vi "Waveform_Generation2.vi"(10 "input cluster":T2) -> (2 "output cluster":T1)   [LabVIEW 2013]
uses:
  waveforms.ctl
  <vilib>/imath/engines/lvmath2/RunTimeEngine/ErrorHandling/NIMS_Finalize Error.vi
  <vilib>/imath/engines/lvmath2/RunTimeEngine/Managers/WorkSpace/UID Generator.vi
  <vilib>/imath/engines/lvmath2/RunTimeEngine/NodeEndStatement/NIMS_NodeEndStatement_Get Vector.vi
  <instcachedir>/0/NIMS_NodeEndStatement_Get Vector_BE4364D373AE46158CA0B14DEB6F98C8.lvgen/NIMS_NodeEndStatement_Get Vector_BE4364D373AE46158CA0B14DEB6F98C8_001.vi
  <vilib>/imath/engines/lvmath/Functions/Error Handling/MergeErrorsWrapper.vi
  <vilib>/imath/engines/lvmath2/RunTimeEngine/Managers/SymbolTable/Clear UID.vi
  <vilib>/imath/engines/lvmath2/RunTimeEngine/NodeEndStatement/NIMS_NodeEndStatement_Output.vi
  <instcachedir>/0/NIMS_NodeEndStatement_Output_53EC0D466D134D7ABD903AC30B43404B.lvgen/NIMS_NodeEndStatement_Output_53EC0D466D134D7ABD903AC30B43404B_011.vi
  <instcachedir>/0/NIMS_NodeEndStatement_Output_53EC0D466D134D7ABD903AC30B43404B.lvgen/NIMS_NodeEndStatement_Output_53EC0D466D134D7ABD903AC30B43404B_001.vi
  <instcachedir>/0/NIMS_NodeEndStatement_Output_53EC0D466D134D7ABD903AC30B43404B.lvgen/NIMS_NodeEndStatement_Output_53EC0D466D134D7ABD903AC30B43404B_005.vi
  <instcachedir>/0/NIMS_NodeEndStatement_Output_53EC0D466D134D7ABD903AC30B43404B.lvgen/NIMS_NodeEndStatement_Output_53EC0D466D134D7ABD903AC30B43404B_010.vi
  <vilib>/imath/engines/lvmath2/RunTimeEngine/RunTimeType/NIMS_RunTimeType_From StrictType (excl LVString).vi
  <instcachedir>/0/NIMS_RunTimeType_From StrictType (excl LVString)_4DEE718D6EB74582AA20236969C084FC.lvgen/NIMS_RunTimeType_From StrictType (excl LVString)_4DEE718D6EB74582AA20236969C084FC_000.vi
  <vilib>/imath/engines/lvmath2/RunTimeEngine/LocalVariableDefStatement/MC_LocalVariableDefStatement_Display.vi
  <vilib>/imath/engines/lvmath2/RunTimeEngine/BuiltInFunctions/abs/NIMS_abs(signed).vi
  <instcachedir>/0/NIMS_abs(signed)_C4FCB8E6058B49B797C7C8D53CA5F6EC.lvgen/NIMS_abs(signed)_C4FCB8E6058B49B797C7C8D53CA5F6EC_000.vi
  <vilib>/imath/engines/lvmath2/RunTimeEngine/BuiltInFunctions/zeros/NIMS_V=zeros(I32,I32).vi
  <vilib>/imathl/engines/lvmath/Functions/Error Handling/Create Error.vi
  <vilib>/imath/engines/lvmath2/RunTimeEngine/RangeToken/NIMS_Range.vi
  <instcachedir>/0/NIMS_Range_7481B155BEE341ECA0F59DDB444E2C09.lvgen/NIMS_Range_7481B155BEE341ECA0F59DDB444E2C09_000.vi
  <vilib>/imath/engines/lvmath2/RunTimeEngine/BuiltInFunctions/linramp/NIMS_linramp.vi
  <vilib>/imath/engines/lvmath2/RunTimeEngine/BuiltInFunctions/length/NIMS_length(GV).vi
  <instcachedir>/0/NIMS_length(GV)_08A3D13377FD4E4B96F5795FBF3698FA.lvgen/NIMS_length(GV)_08A3D13377FD4E4B96F5795FBF3698FA_000.vi
  <vilib>/imath/engines/lvmath2/RunTimeEngine/BuiltInFunctions/repeatmx/NIMS_repeatmx(GM, I32, I32).vi
  <instcachedir>/0/NIMS_repeatmx(GM, I32, I32)_71D32CAC8D434697AB9DA7B55FCB46E4.lvgen/NIMS_repeatmx(GM, I32, I32)_71D32CAC8D434697AB9DA7B55FCB46E4_000.vi
  <vilib>/imath/engines/lvmath2/RunTimeEngine/RowToken/NIMS_RowToken_M_M.vi
  <instcachedir>/0/NIMS_RowToken_M_M_CBE56BFCE95A4183A980645A330616E9.lvgen/NIMS_RowToken_M_M_CBE56BFCE95A4183A980645A330616E9_004.vi
  <vilib>/imath/engines/lvmath2/RunTimeEngine/ErrorHandling/NIMS_Create Error From Enums.vi
  <vilib>/imath/engines/lvmath2/RunTimeEngine/BuiltInFunctions/length/NIMS_length(GM).vi
  <instcachedir>/0/NIMS_length(GM)_47CEC356FCE0482D9BA47DC61C99F2C7.lvgen/NIMS_length(GM)_47CEC356FCE0482D9BA47DC61C99F2C7_000.vi
  <vilib>/imath/engines/lvmath2/RunTimeEngine/IndexRead/NIMS M(S,R2).vi
  <instcachedir>/0/NIMS M(S,R2)_45730E4D0DB74D118F715F4F99DCE4D7.lvgen/NIMS M(S,R2)_45730E4D0DB74D118F715F4F99DCE4D7_000.vi
  <vilib>/imath/engines/lvmath2/RunTimeSupport/NIMS_Error if Not Equal.vi
  <instcachedir>/0/NIMS_Error if Not Equal_902F5D2649E64F5087A1EF57C55C58AB.lvgen/NIMS_Error if Not Equal_902F5D2649E64F5087A1EF57C55C58AB_001.vi
  <vilib>/imath/engines/lvmath2/RunTimeEngine/IndexRead/NIMS V(V).vi
  <instcachedir>/0/NIMS V(V)_298D9CB7BFEB42B8BC8D9C3C28AE8C70.lvgen/NIMS V(V)_298D9CB7BFEB42B8BC8D9C3C28AE8C70_000.vi
  <vilib>/imath/engines/lvmath2/RunTimeEngine/RowToken/NIMS_RowToken_M_SorRV.vi
  <instcachedir>/0/NIMS_RowToken_M_SorRV_6464340A296F47B6970F468C8541F43A.lvgen/NIMS_RowToken_M_SorRV_6464340A296F47B6970F468C8541F43A_000.vi
  <vilib>/imath/engines/lvmath2/RunTimeEngine/RowToken/NIMS_RowToken_SorRV_M.vi
  <instcachedir>/0/NIMS_RowToken_SorRV_M_D0DD9F47061B415B905C482B8C5C3219.lvgen/NIMS_RowToken_SorRV_M_D0DD9F47061B415B905C482B8C5C3219_000.vi
  <vilib>/imath/engines/lvmath2/RunTimeEngine/ArithmeticOperatorToken/NIMS_ArithmeticOperator_plus.vi
  <instcachedir>/0/NIMS_ArithmeticOperator_plus_8A46DAFC24D445C9B2C97B626139369E.lvgen/NIMS_ArithmeticOperator_plus_8A46DAFC24D445C9B2C97B626139369E_003.vi
  <vilib>/imath/engines/lvmath2/RunTimeEngine/BuiltInFunctions/round/NIMS_round(DBL-S).vi
  <vilib>/imath/engines/lvmath2/RunTimeEngine/BuiltInFunctions/ones/NIMS_V=ones(I32,I32).vi
  <instcachedir>/0/NIMS_repeatmx(GM, I32, I32)_71D32CAC8D434697AB9DA7B55FCB46E4.lvgen/NIMS_repeatmx(GM, I32, I32)_71D32CAC8D434697AB9DA7B55FCB46E4_004.vi
  <instcachedir>/0/NIMS_RowToken_M_M_CBE56BFCE95A4183A980645A330616E9.lvgen/NIMS_RowToken_M_M_CBE56BFCE95A4183A980645A330616E9_005.vi
  <vilib>/imath/engines/lvmath2/RunTimeEngine/RangeToken/NIMS_Range_R2 - Integer.vi
  <instcachedir>/0/NIMS_Range_R2 - Integer_C51C130E5EA5464EA148B28CDAB9615A.lvgen/NIMS_Range_R2 - Integer_C51C130E5EA5464EA148B28CDAB9615A_000.vi
  <vilib>/imath/engines/lvmath2/RunTimeEngine/CommandStatement/MC_CommandStatement_break.vi
  <vilib>/imath/engines/lvmath2/RunTimeEngine/ArithmeticOperatorToken/NIMS_ArithmeticOperator_power(S).vi
  <instcachedir>/0/NIMS_ArithmeticOperator_power(S)_7602F12E697C47D8910FAD43BB85D848.lvgen/NIMS_ArithmeticOperator_power(S)_7602F12E697C47D8910FAD43BB85D848_011.vi
  <instcachedir>/0/NIMS_ArithmeticOperator_plus_8A46DAFC24D445C9B2C97B626139369E.lvgen/NIMS_ArithmeticOperator_plus_8A46DAFC24D445C9B2C97B626139369E_004.vi
  <vilib>/imath/engines/lvmath2/RunTimeEngine/BuiltInFunctions/difference/NIMS_difference(GV,I32).vi
  <instcachedir>/0/NIMS_difference(GV,I32)_DC7351DCBCF840A8AE147F50EC2CE86E.lvgen/NIMS_difference(GV,I32)_DC7351DCBCF840A8AE147F50EC2CE86E_000.vi
  <vilib>/imath/engines/lvmath2/RunTimeEngine/VariableToken/Support/NIMS_Vector Boolean Index to I32 Index.vi
  <vilib>/imath/engines/lvmath2/RunTimeEngine/IndexReplace/NIMS V(V)=V.vi
  <instcachedir>/0/NIMS V(V)=V_320D50C59D214ECA9A3F84A49F4F0CE6.lvgen/NIMS V(V)=V_320D50C59D214ECA9A3F84A49F4F0CE6_000.vi
  <vilib>/imath/engines/lvmath2/RunTimeEngine/IndexRead/NIMS V(R2).vi
  <instcachedir>/0/NIMS V(R2)_C76619605A0E4E9F8B2FA9389712AC47.lvgen/NIMS V(R2)_C76619605A0E4E9F8B2FA9389712AC47_000.vi
  <vilib>/imath/engines/lvmath2/RunTimeEngine/BuiltInFunctions/quadn_trap/NIMS_quadn_trap(GV).vi
  <instcachedir>/0/NIMS_quadn_trap(GV)_FA03A60467B0476FA3B590A5FD2D65B5.lvgen/NIMS_quadn_trap(GV)_FA03A60467B0476FA3B590A5FD2D65B5_000.vi
  <vilib>/imath/engines/lvmath2/RunTimeEngine/IndexReplace/NIMS V(S)=S.vi
  <instcachedir>/0/NIMS V(S)=S_66A18068148B4981A312229A93EA5C06.lvgen/NIMS V(S)=S_66A18068148B4981A312229A93EA5C06_000.vi
  <vilib>/imath/engines/lvmath2/RunTimeEngine/BuiltInFunctions/min/1 input/NIMS_min(RV).vi
  <instcachedir>/0/NIMS_min(RV)_EE2DD3E2888846108C5160A664B67832.lvgen/NIMS_min(RV)_EE2DD3E2888846108C5160A664B67832_000.vi
  <vilib>/imath/engines/lvmath2/RunTimeEngine/IndexReplace/NIMS V(V)=S.vi
  <instcachedir>/0/NIMS V(V)=S_43E6004D39A2403BA86EB2871913A93B.lvgen/NIMS V(V)=S_43E6004D39A2403BA86EB2871913A93B_000.vi
  <vilib>/imath/engines/lvmath2/RunTimeEngine/Managers/SymbolTable/NIMS_WorkSpace.lvlib
panel:
  out "output waveform":digitaldata
  out "analog waveform array dev2":waveform(dbl)[](array[waveform])
  out "analog waveform array":waveform(dbl)[](array[waveform])
  out "laser":i32
  out "Lens2":waveform(dbl)(graph)
  out "Lens1":waveform(dbl)(graph)
  out "Piezo":waveform(dbl)(graph)
  out "Camera":digitalwaveform(graph)
  out "Z_mirror":waveform(dbl)(graph)
  out "Scan mirror":waveform(dbl)(graph)
  out "waveform_length":i32
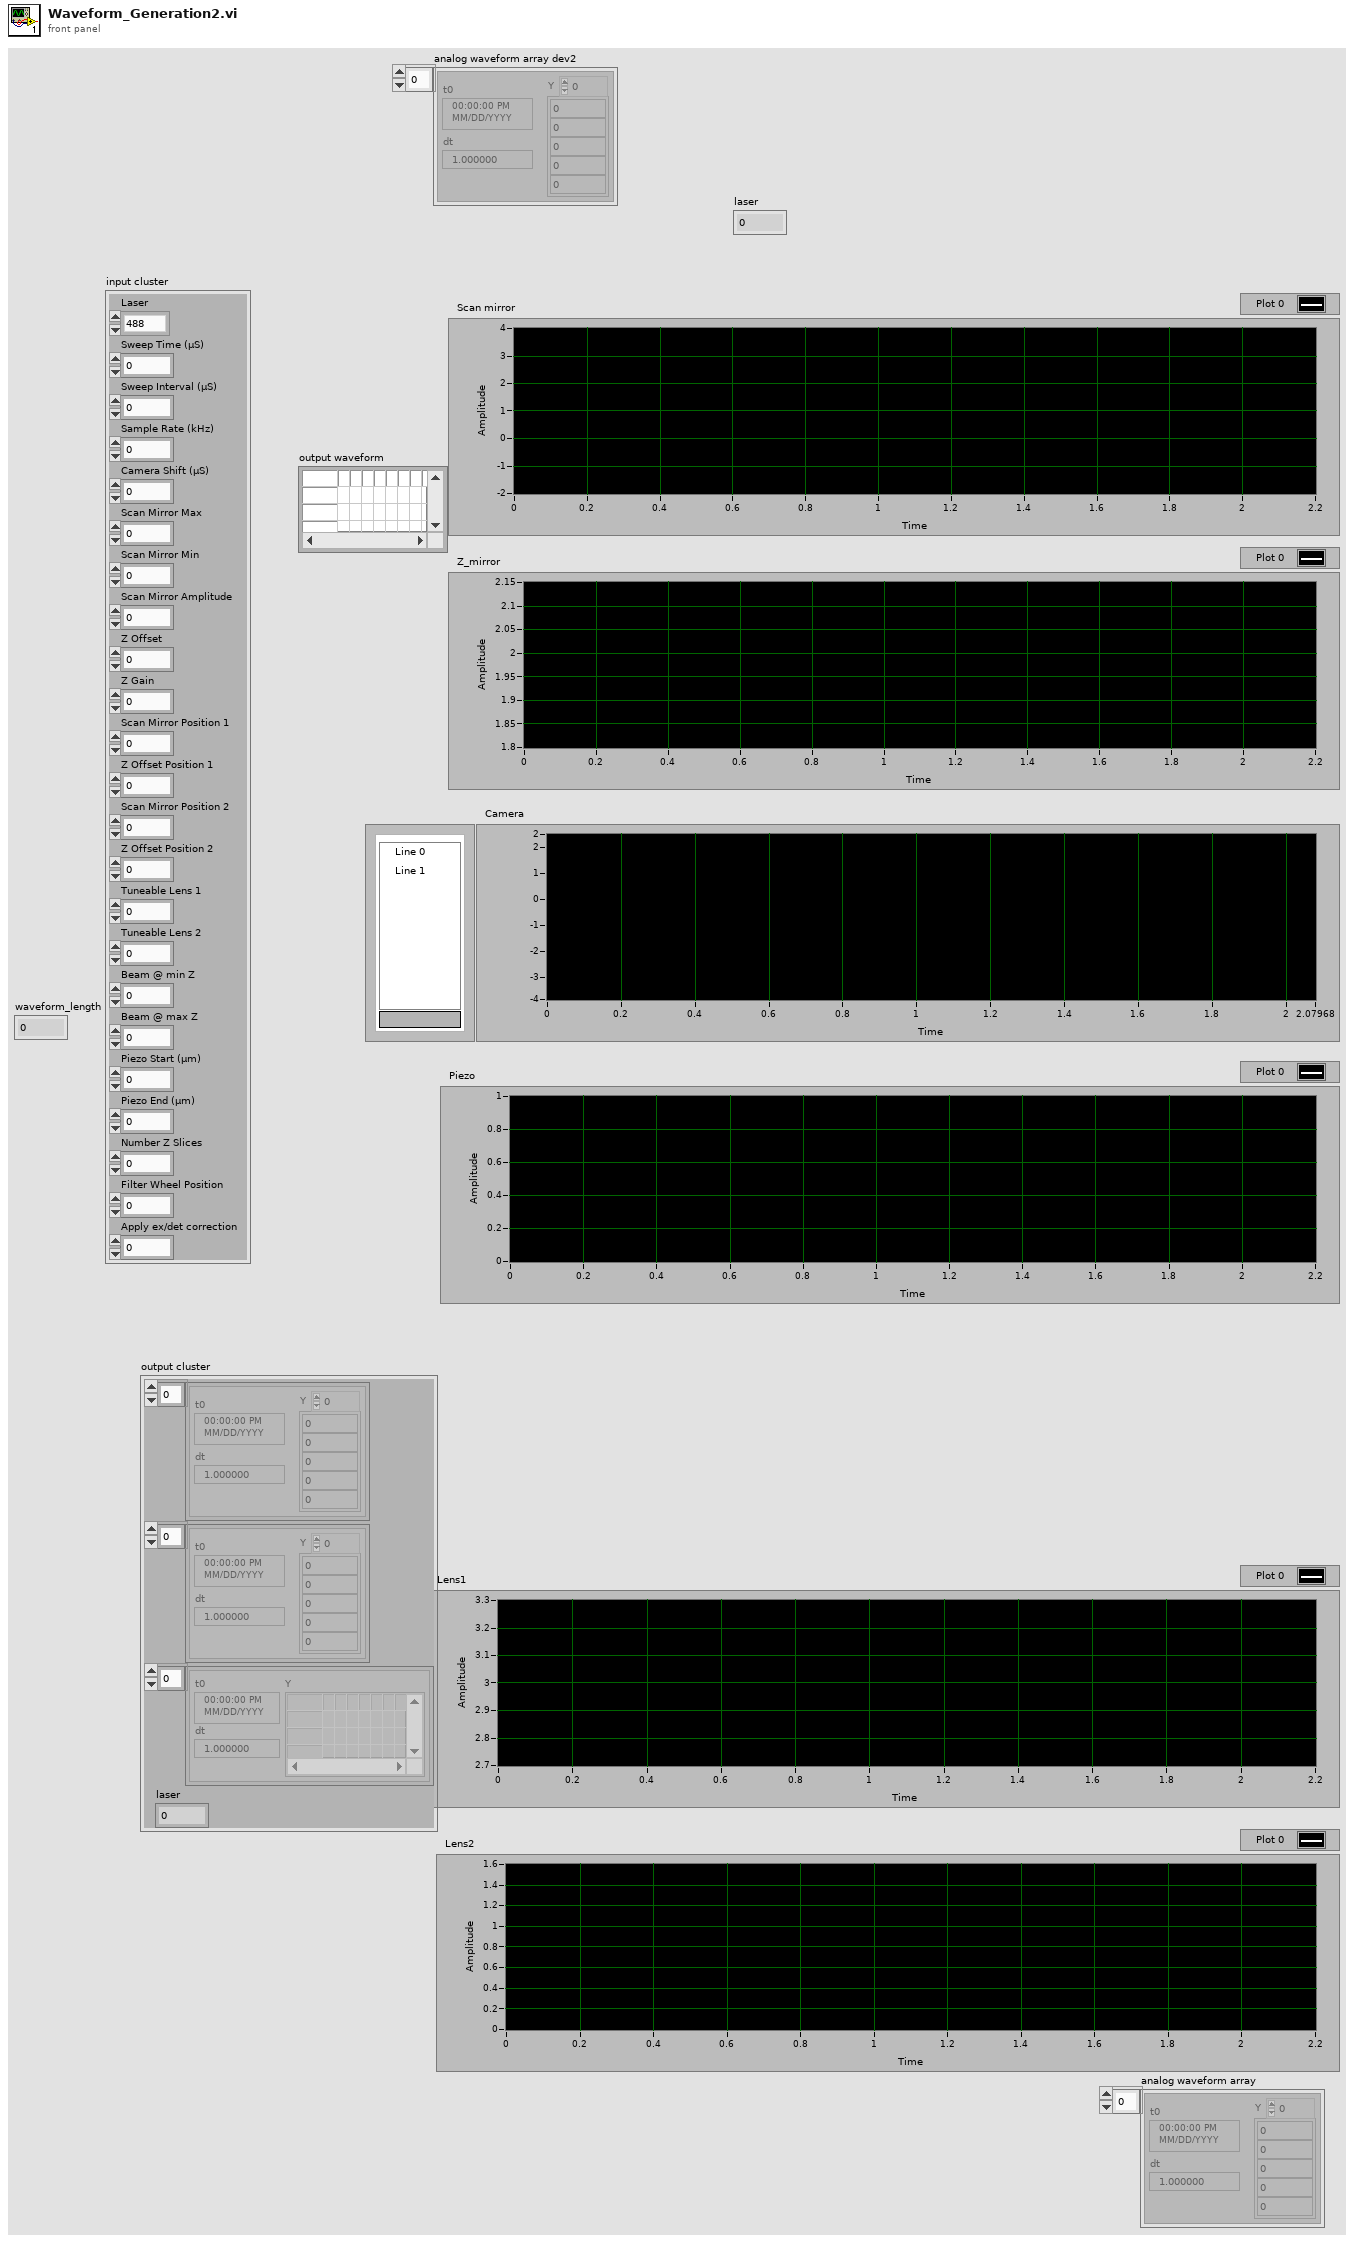
[diagram p1: front panel]
types:
  T1 = typedef "waveforms.ctl" = cluster{waveform(dbl)[], waveform(dbl)[], digitalwaveform[], "laser":i32}
  T2 = cluster{"Laser":enum16{"488", "561"}, "Sweep Time (µS)":u32, "Sweep Interval (µS)":u32, "Sample Rate (kHz)":dbl, "Camera Shift (µS)":dbl, "Scan Mirror Max":dbl, "Scan Mirror Min":dbl, "Scan Mirror Amplitude":dbl, "Z Offset":dbl, "Z Gain":dbl, "Scan Mirror Position 1":dbl, "Z Offset Position 1":dbl, "Scan Mirror Position 2":dbl, "Z Offset Position 2":dbl, "Tuneable Lens 1":dbl, "Tuneable Lens 2":dbl, "Beam @ min Z":dbl, "Beam @ max Z":dbl, "Piezo Start (µm)":dbl, "Piezo End (µm)":dbl, "Number Z Slices":i16, "Filter Wheel Position":i32, "Apply ex/det correction":u16}
  T3 = cluster{waveform(dbl)[], waveform(dbl)[], digitalwaveform[], "laser":i32}
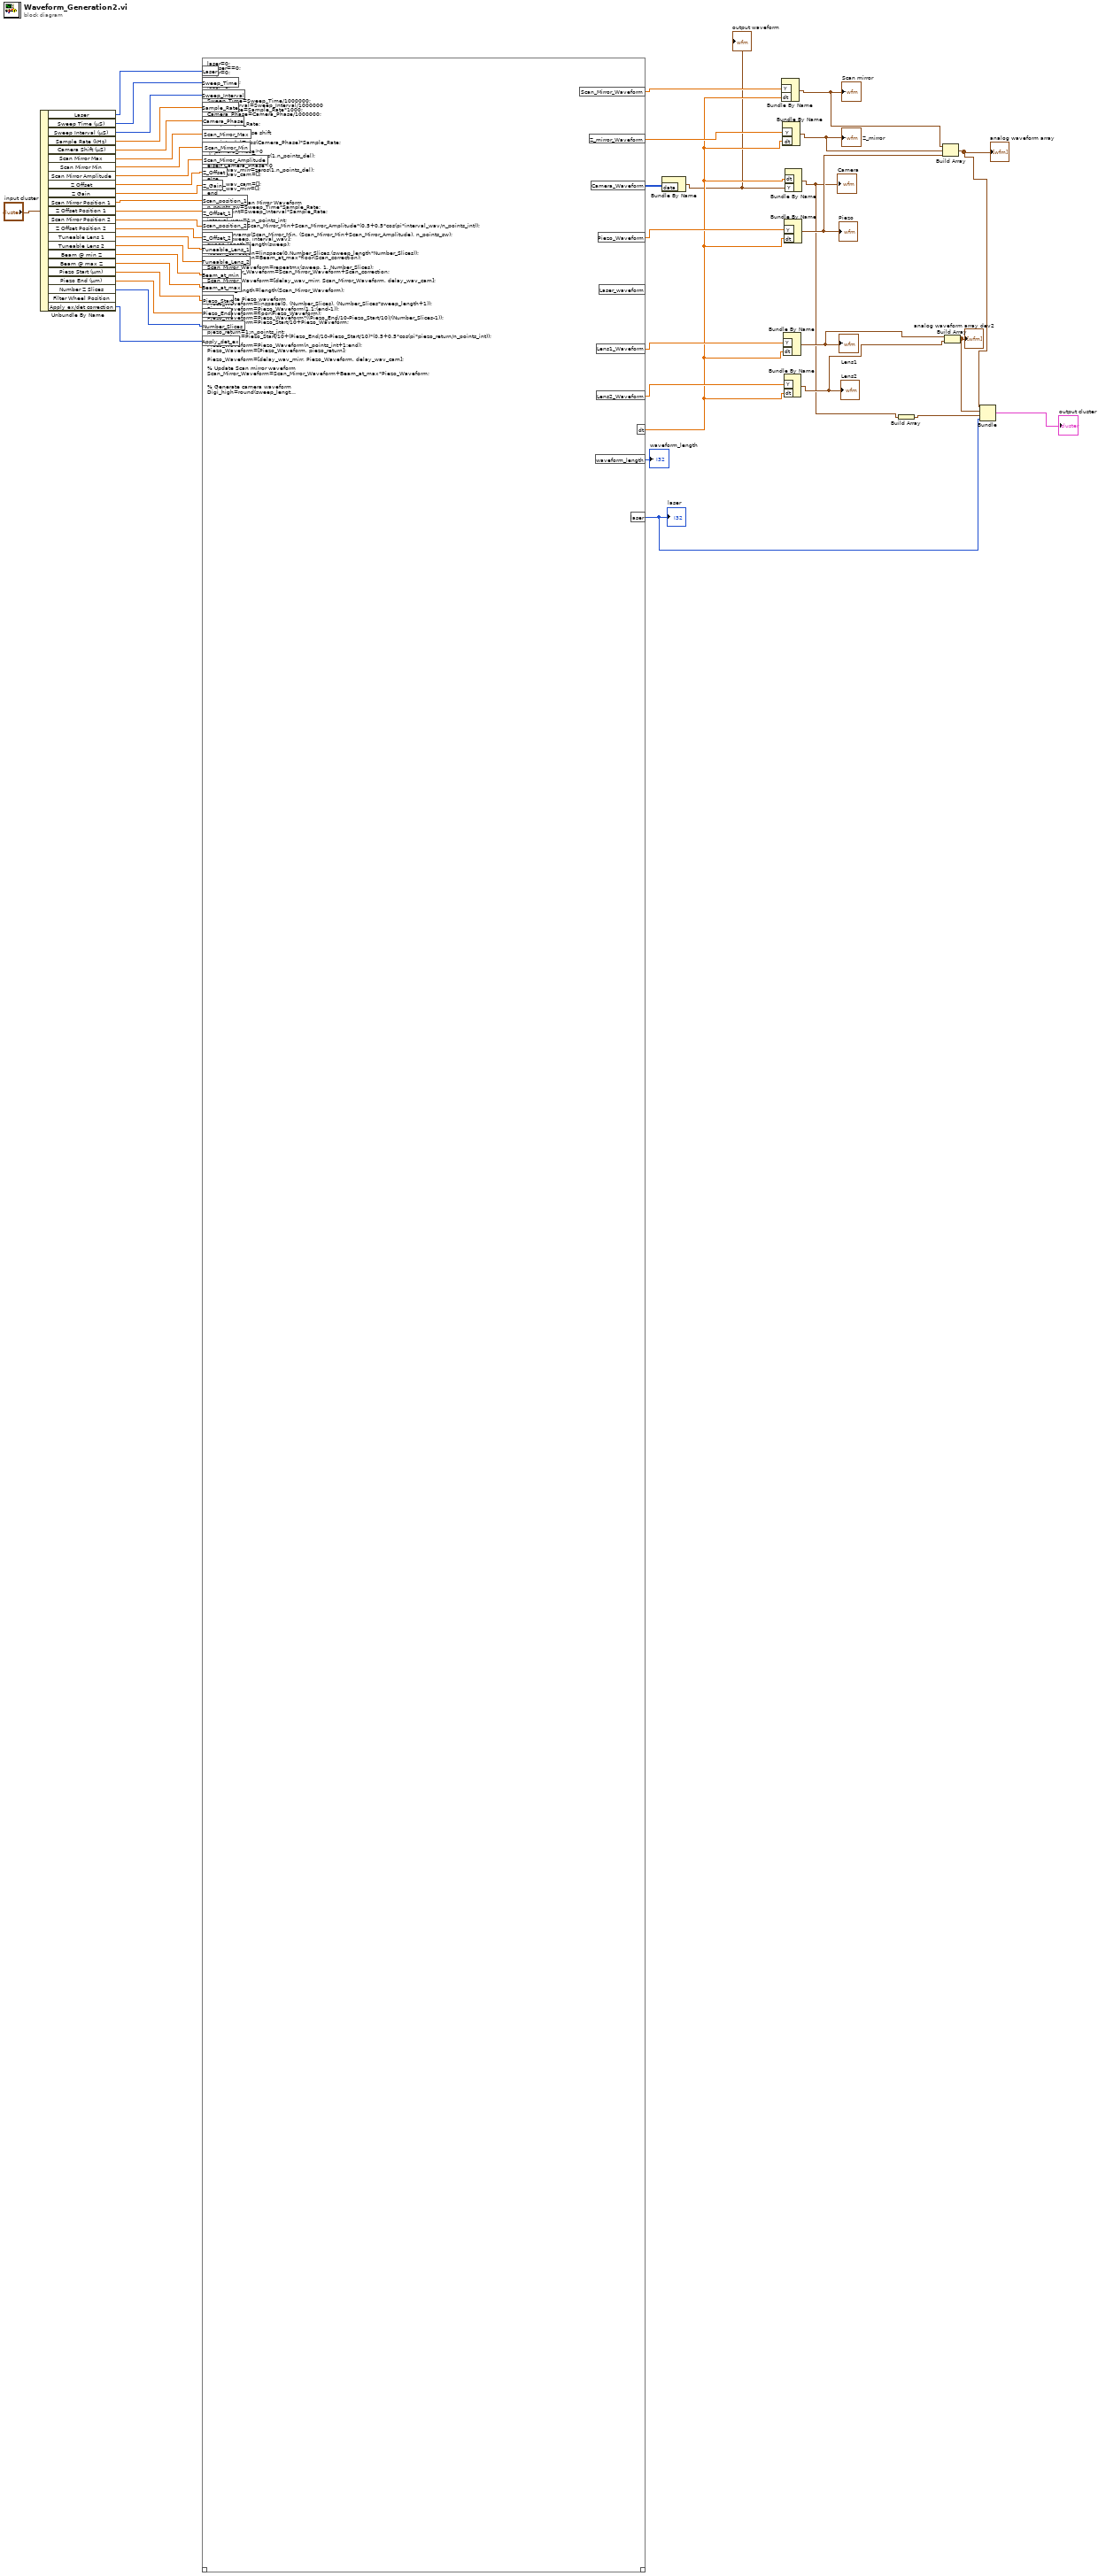
[diagram p0: block diagram]
diagram:
  n1 = Unbundle By Name("input cluster") -> ("Laser"=w43:enum16{"488", "561"}, "Sweep Time (µS)"=w42:u32, "Sweep Interval (µS)"=w41:u32, "Sample Rate (kHz)"=w40:dbl, "Camera Shift (µS)"=w39:dbl, "Scan Mirror Max"=w38:dbl, "Scan Mirror Min"=w37:dbl, "Scan Mirror Amplitude"=w36:dbl, "Z Offset"=w35:dbl, "Z Gain"=w34:dbl, "Scan Mirror Position 1"=w33:dbl, "Z Offset Position 1"=w32:dbl, "Scan Mirror Position 2"=w31:dbl, "Z Offset Position 2"=w30:dbl, "Tuneable Lens 1"=w29:dbl, "Tuneable Lens 2"=w28:dbl, "Beam @ min Z"=w27:dbl, "Beam @ max Z"=w26:dbl, "Piezo Start (µm)"=w25:dbl, "Piezo End (µm)"=w24:dbl, "Number Z Slices"=w23:i16, "Apply ex/det correction"=w22:u16)  [unwired: 1 out]
  n2 = mathscript code="laser=0;\nif Laser==0;\nlaser=0;\nend\nif Laser==1;\nlaser=1;\nend\n\nSweep_Time=Sweep_Time/1000000;\nSweep_Interval=Sweep_Interval/1000000\nSample_Rate=Sample_Rate*1000;\nCamera_Phase=Camera_Phase/1000000;\n\ndt=1/Sample_Rate;\n\n% Establish phase shift\n\nn_points_del=abs(Camera_Phase)*Sample_Rate;\n\n if Camera_Phase>0\ndelay_wav_cam=zeros(1,n_points_del);\ndelay_wav_mirr=[];\nelseif Camera_Phase<0\ndelay_wav_mirr=zeros(1,n_points_del);\ndelay_wav_cam=[];\nelse\ndelay_wav_cam=[];\ndelay_wav_mirr=[];\nend\n\n% Generate Scan Mirror Waveform\nn_points_sw=Sweep_Time*Sample_Rate;\nn_points_int=Sweep_Interval*Sample_Rate;\n\ninterval_wav=1:n_points_int;\ninterval_wav=Scan_Mirror_Min+Scan_Mirror_Amplitude*(0.5+0.5*cos(pi*interval_wav/n_points_int));\n\nsweep=linramp(Scan_Mirror_Min, (Scan_Mirror_Min+Scan_Mirror_Amplitude), n_points_sw);\nsweep=[sweep, interval_wav];\nsweep_length=length(sweep);\n\n%Scan_correction=linspace(0,Number_Slices,(sweep_length*Number_Slices));\n%Scan_correction=Beam_at_max*floor(Scan_correction);\n\nScan_Mirror_Waveform=repeatmx(sweep, 1, Number_Slices);\n%Scan_Mirror_Waveform=Scan_Mirror_Waveform+Scan_correction;\n\nScan_Mirror_Waveform=[delay_wav_mirr, Scan_Mirror_Waveform, delay_wav_cam];\n\nwaveform_length=length(Scan_Mirror_Waveform);\n\n% Generate Piezo waveform\nPiezo_Waveform=linspace(0, (Number_Slices), (Number_Slices*sweep_length+1));\nPiezo_Waveform=Piezo_Waveform(1,1:(end-1));\nPiezo_Waveform=floor(Piezo_Waveform);\nPiezo_Waveform=Piezo_Waveform*((Piezo_End/10-Piezo_Start/10)/(Number_Slices-1));\nPiezo_Waveform=Piezo_Start/10+Piezo_Waveform;\n\npiezo_return=1:n_points_int;\npiezo_return=Piezo_Start/10+(Piezo_End/10-Piezo_Start/10)*(0.5+0.5*cos(pi*piezo_return/n_points_int));\n\nPiezo_Waveform=Piezo_Waveform(n_points_int+1:end);\nPiezo_Waveform=[Piezo_Waveform, piezo_return];\n\nPiezo_Waveform=[delay_wav_mirr, Piezo_Waveform, delay_wav_cam];\n\n% Update Scan mirror waveform\nScan_Mirror_Waveform=Scan_Mirror_Waveform+Beam_at_max*Piezo_Waveform;\n\n\n% Generate camera waveform\nDigi_high=round(sweep_length/10);\nDigi_low=sweep_length-Digi_high;\n\nCamera_Waveform=[ones(1,Digi_high) zeros(1,Digi_low)];\nCamera_Waveform=repeatmx(Camera_Waveform,1,Number_Slices);\nCamera_Waveform=[delay_wav_cam, Camera_Waveform, delay_wav_mirr]';\n\n% Generate Z_mirror\nZ_mirror_Waveform=Z_Offset+Z_Gain*Piezo_Waveform;\nex_det_corr=[linramp(-Z_Offset_2/2,Z_Offset_2/2,n_points_sw), zeros(1,n_points_int)];\nex_det_corr=repeatmx(ex_det_corr,1,Number_Slices);\nex_det_corr=[delay_wav_mirr, ex_det_corr, delay_wav_cam];\n\nZ_mirror_Waveform=Z_mirror_Waveform+ex_det_corr;\n\n% Generate laser\nLaser_waveform=[ones(1,n_points_sw), zeros(1,n_points_int)];\nLaser_waveform=repeatmx(Laser_waveform,1,Number_Slices);\nLaser_waveform=[delay_wav_mirr, Laser_waveform, delay_wav_cam]';\n\n% Generate lens 1 waveform\n  Lens1_Waveform=Tuneable_Lens_1*ones(1,waveform_length);\n   %Lens1_Waveform=Scan_Mirror_Waveform;\n   %Lens1_Waveform=linspace(Tuneable_Lens_1,Tuneable_Lens_1+0.3,waveform_length)\n\n% bent switch\nbent_state =Z_Offset_1;\n\n%%%%%%%%%%%%%%%%%%%%%%%%% static\nif bent_state ==0\n\n% Generate lens 2 waveform\n   Lens1_Waveform=Tuneable_Lens_1*ones(1,waveform_length);\n   Lens2_Waveform=Tuneable_Lens_2*ones(1,waveform_length);\n\n   %Lens2_Waveform=0.5*cos(linspace(-pi/2,pi/2,n_points_sw))+0.5;\n   %Lens2_Waveform=Lens2_Waveform*2+Tuneable_Lens_2;\n   %Lens2_Waveform=[Lens2_Waveform, Tuneable_Lens_2*ones(1,n_points_int)];\n   %Lens2_Waveform=repeatmx(Lens2_Waveform,1,Number_Slices);\n   %Lens2_Waveform=[delay_wav_cam, Lens2_Waveform, delay_wav_mirr];\n\n\n%%%%%%%%%%%%%%%%%%%%%%%%% \nelseif  bent_state ==2\n\nLens2_Waveform=Tuneable_Lens_2*ones(1,waveform_length);\n\nR=Scan_position_1;\noffset=0.0;\nCorr=0;\n\nLens1_Waveform=[];\n\nfor n=0:Number_Slices-1\nLens1_sweep=Tuneable_Lens_1*ones(1,sweep_length);\n    \nb=R*sqrt(1-((Number_Slices-n)/Number_Slices)^2);    \na=sqrt(1-((Number_Slices-n)/Number_Slices)^2);\n\nX=linspace(-1,1,(n_points_sw-2*floor(offset*n_points_sw)));\nY=b*sqrt(1-(X./a).^2);\nY=real(Y);\n\nY=Y+Corr*linspace(0,100,length(Y));\nY=[zeros(1,floor(offset*n_points_sw)),Y,zeros(1,floor(offset*n_points_sw)),zeros(1,n_points_int)];\n\nLens1_sweep=Lens1_sweep + Y;\n\nLens1_Waveform=[Lens1_Waveform, Lens1_sweep];\n\n\nend\n\nLens1_Waveform=[delay_wav_mirr, Lens1_Waveform, delay_wav_cam];\n\n%%%%%%%%%%%%%%%%%%%%\n\nelseif bent_state==3\n\nR=Scan_position_1;\nY=Scan_position_2;\n\nLens1_Waveform=Tuneable_Lens_1*ones(1,waveform_length);\n\nLens2_wav=Tuneable_Lens_2*ones(1,n_points_sw-round(0.9*n_points_sw));\nLens2_wav2=Tuneable_Lens_2+R*linspace(0,1,round(0.9*n_points_sw));\nLens2_wav2(Lens2_wav2>Y)=Y;\n\nLens2_Waveform=[Lens2_wav, Lens2_wav2, Tuneable_Lens_2*ones(1,n_points_int)];\nLens2_Waveform=repeatmx(Lens2_Waveform,1,Number_Slices);\nLens2_Waveform=[delay_wav_mirr, Lens2_Waveform, delay_wav_cam];\n\n%%%%%%%%%%%%%%%%%%%%%\n\nelseif bent_state==4\n\nR=Scan_position_1;\nY=Scan_position_2;\n\nLens1_Waveform=Tuneable_Lens_1*ones(1,waveform_length);\n\nX=linspace(-2,4,n_points_sw);\n\nLens2_wav=exp(-R*X);\nLens2_wav2=Tuneable_Lens_2+Y*((1+Lens2_wav).^-1);\n\nXint=linspace(2,-4,n_points_int);\n\nLens2_wavint=exp(-R*Xint);\nLens2_wav2int=Tuneable_Lens_2+Y*((1+Lens2_wavint).^-1);\n\nLens2_Waveform=[Lens2_wav2, Lens2_wav2int];\nLens2_Waveform=repeatmx(Lens2_Waveform,1,Number_Slices);\nLens2_Waveform=[delay_wav_mirr, Lens2_Waveform, delay_wav_cam];\n\n%%%%%%%%%%%%%%%%%%\n\nelseif bent_state==5\n\nR=Scan_position_1;\nY=Scan_position_2;\n\nLens1_Waveform=Tuneable_Lens_1*ones(1,waveform_length);\n\nX=linspace(0,2*pi,n_points_sw);\n\nLens2_wav2=Y*sin(R*X);\n\nLens2_Waveform=[Lens2_wav2, Tuneable_Lens_2*ones(1,n_points_int)];\nLens2_Waveform=repeatmx(Lens2_Waveform,1,Number_Slices);\nLens2_Waveform=[delay_wav_mirr, Lens2_Waveform, delay_wav_cam];\n\n%%%%%%%%%%%%%%%%%%\n\nelseif bent_state==6\n\nR=Scan_position_1;\nY=Scan_position_2;\n\nLens1_Waveform=Tuneable_Lens_1*ones(1,waveform_length);\n\nLens_wav1=Tuneable_Lens_2+R*linspace(0,1,round(n_points_sw/2));\nLens_wav2=Tuneable_Lens_2+R*linspace(1,0,n_points_sw-round(n_points_sw/2))\n\nLens2_Waveform=[Lens_wav1, Lens_wav2, Tuneable_Lens_2*ones(1,n_points_int)];\nLens2_Waveform=repeatmx(Lens2_Waveform,1,Number_Slices);\nLens2_Waveform=[delay_wav_mirr, Lens2_Waveform, delay_wav_cam];\n\n%%%%%%%%%%%%%%%%%%%%%%%\n\nelseif bent_state==7\n\nLens1_Waveform=Tuneable_Lens_1*ones(1,waveform_length);\nLens2_sweep=Tuneable_Lens_2*ones(1,sweep_length);\n\nR=Scan_position_1;\noffset1=0;\noffset2=0.3;\nfac=Beam_at_min;\nfac2=Scan_position_2;\n\nx=linspace(-1,1,(n_points_sw-floor(offset1*n_points_sw)-floor(offset2*n_points_sw)));;\ny=R*cos(x*pi);\n%y=R*real(sqrt(1-x.^2));\nyp=fac2*diff(y);\nyp(yp<0)=fac*yp(yp<0);\n\nyi=zeros(1,length(x)-1);\nfor i=1:(length(x)-1)\nyi(i)=trapz(yp(1:i));\nend\n\nyi=[0,zeros(1,floor(offset1*n_points_sw)),yi,min(yi)*ones(1,floor(offset2*n_points_sw)),zeros(1,n_points_int)];\n\nLens2_sweep=Lens2_sweep + yi;\n\nLens2_Waveform=repeatmx(Lens2_sweep,1,Number_Slices);\n\nLens2_Waveform=[delay_wav_mirr, Lens2_Waveform, delay_wav_cam];\n\n%%%%%%%%%%%%%%%%%%\n\nelseif bent_state==8\n\nLens1_Waveform=Tuneable_Lens_1*ones(1,waveform_length);\nLens2_sweep=Tuneable_Lens_2*ones(1,sweep_length);\n\nR=Scan_position_1;\noffset=0.4;\nfac2=Scan_position_2;\nfac=Beam_at_min;\n\nx=linspace(-1,1,n_points_sw);\ny=R*cos(x*pi);\n%y=R*real(sqrt((1-offset)^2-x.^2));\nyp=fac2*diff(y);\nyp(yp<0)=fac*yp(yp<0);\n\nyi=zeros(1,length(x)-1);\nfor i=1:(length(x)-1)\nyi(i)=trapz(yp(1:i));\nend\n\nyi=[0,yi,zeros(1,n_points_int)];\n\nLens2_sweep=Lens2_sweep + yi;\n\nLens2_Waveform=repmat(Lens2_sweep,1,Number_Slices);\n\nLens2_Waveform=[delay_wav_mirr, Lens2_Waveform, delay_wav_cam];\n\n%%%%%%%%%%%%%%%%%% multiple sinusioids\n\nelseif bent_state==9\n\nR=Scan_position_1;\nfreq=100*Scan_position_2;\n\nLens1_Waveform=Tuneable_Lens_1*ones(1,waveform_length);\n\nLens2_sweep=Tuneable_Lens_2*ones(1,sweep_length);\n\nx=linspace(-pi,pi,n_points_sw);\ny=Tuneable_Lens_2+0.5*R*(1+cos(x*freq));\ny=[y,Tuneable_Lens_2*ones(1,n_points_int)]\n\nLens2_Waveform=repmat(y,1,Number_Slices);\nLens2_Waveform=[delay_wav_mirr, Lens2_Waveform, delay_wav_cam];\n\n%%%%%%%%%%%%%%%%%% multiple sinusioids reversed\n\nelseif bent_state==10\n\nR=Scan_position_1;\nfreq=100*Scan_position_2;\n\nLens1_Waveform=Tuneable_Lens_1*ones(1,waveform_length);\n\nLens2_sweep=Tuneable_Lens_2*ones(1,sweep_length);\n\nx=linspace(-pi,pi,n_points_sw);\ny=Tuneable_Lens_2+0.5*R*(1-cos(x*freq));\ny=[y,(Tuneable_Lens_2+R)*ones(1,n_points_int)]\n\nLens2_Waveform=repmat(y,1,Number_Slices);\nLens2_Waveform=[delay_wav_mirr, Lens2_Waveform, delay_wav_cam];\n\n%%%%%%%%%%%%%%%%%%\n\n%%%%%%%%%%%%%%%%%%\nelse\nLens1_Waveform=Tuneable_Lens_1*ones(1,waveform_length);\n\nR=Scan_position_1;\noffset=0.0;\nCorr=Scan_position_2;;\n\nLens2_Waveform=[];\n\nfor n=0:Number_Slices-1\nLens2_sweep=Tuneable_Lens_2*ones(1,sweep_length);\n    \nb=R*sqrt(1-((Number_Slices-n)/Number_Slices)^2);    \na=sqrt(1-((Number_Slices-n)/Number_Slices)^2);\n\nX=linspace(-1,1,(n_points_sw-2*floor(offset*n_points_sw)));\nY=b*sqrt(1-(X./a).^2);\nY=real(Y);\n\nY=Y+Corr*linspace(0,1,length(Y));\nY=[zeros(1,floor(offset*n_points_sw)),Y,zeros(1,floor(offset*n_points_sw)),zeros(1,n_points_int)];\n\nLens2_sweep=Lens2_sweep + Y;\n\nLens2_Waveform=[Lens2_Waveform, Lens2_sweep];\n\n\nend\n\nLens2_Waveform=[delay_wav_mirr, Lens2_Waveform, delay_wav_cam];\n\nend\n\n\n%Combine digital waveforms\nCamera_Waveform=[Camera_Waveform, Laser_waveform];"("Laser"=w43, "Sweep_Time"=w42, "Sweep_Interval"=w41, "Sample_Rate"=w40, "Camera_Phase"=w39, "Scan_Mirror_Max"=w38, "Scan_Mirror_Min"=w37, "Z_Offset"=w35, "Scan_Mirror_Amplitude"=w36, "Z_Gain"=w34, "Scan_position_1"=w33, "Z_Offset_2"=w30, "Z_Offset_1"=w32, "Scan_position_2"=w31, "Tuneable_Lens_1"=w29, "Tuneable_Lens_2"=w28, "Beam_at_min"=w27, "Beam_at_max"=w26, "Piezo_Start"=w25, "Piezo_End"=w24, "Number_Slices"=w23, "Apply_det_ex"=w22) -> ("Scan_Mirror_Waveform"=w19:dbl[], "Z_mirror_Waveform"=w18:dbl[], "Piezo_Waveform"=w17:dbl[], "Camera_Waveform"=w21:i32[][], "Lens1_Waveform"=w16:dbl[], "Lens2_Waveform"=w15:dbl[], "dt"=w14:dbl, "waveform_length"=→"waveform_length":i32, "laser"=w5:i32)  [unwired: 1 in, 2 out]
  "laser" <- w5
  n3 = Bundle By Name("data"=w21) -> (w4:digitaldata)  [unwired: 1 in]
  "output waveform" <- w4
  n4 = Bundle By Name ("Build Waveform")("Y"=w19, "dt"=w14) -> (w12:waveform(dbl))  [unwired: 1 in]
  "Scan mirror" <- w12
  n5 = Bundle By Name("Y"=w18, "dt"=w14) -> (w11:waveform(dbl))  [unwired: 1 in]
  "Z_mirror" <- w11
  n6 = Bundle By Name("Y"=w16, "dt"=w14) -> (w9:waveform(dbl))  [unwired: 1 in]
  "Lens1" <- w9
  n7 = Bundle By Name("Y"=w15, "dt"=w14) -> (w8:waveform(dbl))  [unwired: 1 in]
  "Lens2" <- w8
  n8 = Bundle By Name("Y"=w17, "dt"=w14) -> (w10:waveform(dbl))  [unwired: 1 in]
  "Piezo" <- w10
  n9 = Bundle By Name("dt"=w14, "Y"=w4) -> (w2:digitalwaveform)  [unwired: 1 in]
  "Camera" <- w2
  n10 = Build Array(w2) -> (w1:digitalwaveform[])
  n11 = Build Array(w12, w11, w10) -> (w7:waveform(dbl)[])
  "analog waveform array" <- w7
  n12 = Build Array(w9, w8) -> (w6:waveform(dbl)[])
  "analog waveform array dev2" <- w6
  n13 = Bundle(w7, w6, w1, "laser"=w5) -> (→"output cluster":T3)  [unwired: 1 in]
